vi "Read Pass_.vi"(8 "error in (no error)":errorcluster, 11 "BallInterception in":refnum<class "BallInterception.lvclass">) -> (0 "error out":errorcluster, 2 "Pass?":bool, 3 "BallInterception out":refnum<class "BallInterception.lvclass">)   [LabVIEW 2023, in "BallInterception.lvclass"]
uses:
  BallInterception.lvclass
  BallInterception.lvclass/BallInterception.ctl
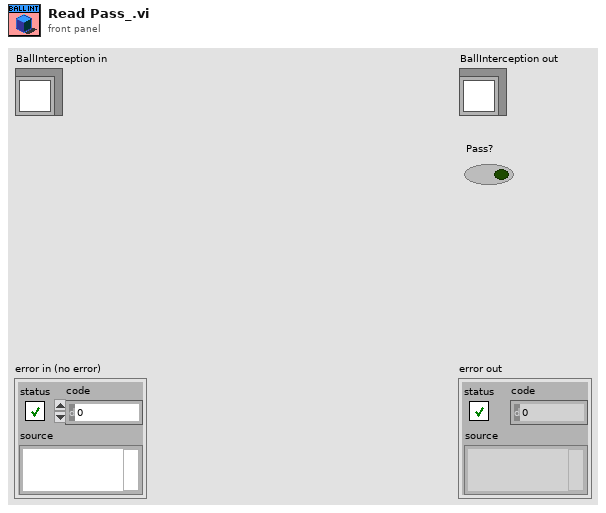
[diagram p1: front panel]
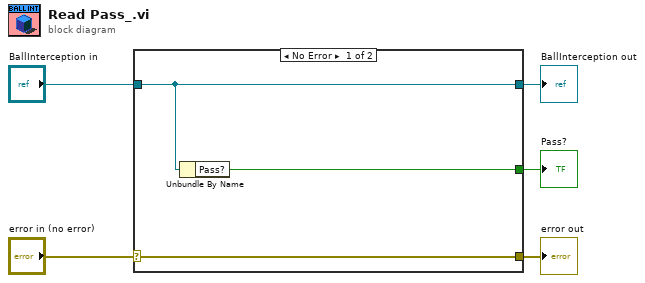
[diagram p0: block diagram]
diagram:
  n1 = case shown="No Error" "error in (no error)" {
    selector: "error in (no error)" -> [w8 w9]
    tunnel: [w8 w9] -> w4
    tunnel: [w7 w10] -> w2
    tunnel: "BallInterception in" -> [w7 w10]
    tunnel: [w6 _] -> w1
    frame No Error {
      n2 = Unbundle By Name(w7) -> ("Pass?"=w6:bool)
    }
    frame Error {
    }
  }
  "error out" <- w4
  "BallInterception out" <- w2
  "Pass?" <- w1
